vi "peakFinder.vi"(11 "Input Signal":dbl[](array[numeric])) -> (2 "Peak Index":i32, 3 "Half Max Height":dbl)   [LabVIEW 2016]
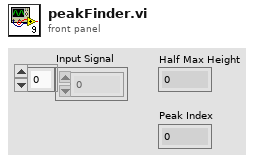
[diagram p1: front panel]
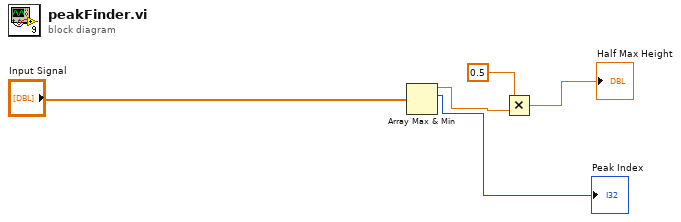
[diagram p0: block diagram]
diagram:
  n1 = Array Max & Min(array="Input Signal") -> (max value=w3:dbl, max index (indices)=→"Peak Index":i32)  [unwired: 2 out]
  n2 = Multiply(x=0.5, y=w3) -> (x*y=→"Half Max Height":dbl)
